vi "Prosilica Oscillating Exp.vi"() -> ()   [LabVIEW 2011]
uses:
  <vilib>/userDefined/High Color/IMAQdx.ctl
  <vilib>/vision/driver/IMAQdx.llb/IMAQdx Acquisition Mode.ctl
  <vilib>/vision/driver/IMAQdx.llb/IMAQdx Buffer Number Mode.ctl
  <vilib>/Platform/TimedLoop/XDataNode/timing_clust.ctl
  <vilib>/Platform/TimedLoop/XDataNode/nitl_modes.ctl
  <vilib>/Platform/TimedLoop/XDataNode/wakeup.ctl
  <vilib>/Platform/TimedLoop/XDataNode/XDataNode.xnode
  Program Files/National Instruments/LabVIEW 2011/resource/objmgr/imaqdx.rc
  <vilib>/vision/driver/NI_Vision_Acquisition_Software.lvlib
  Program Files/Mad City Labs/NanoDrive/Madlib.dll
  <vilib>/Platform/TimedLoop/XDataNode/XDNodeRunTimeDep.lvlib
panel:
  out "Starting Temperature":dbl
  out "Sample=Setpoints!":bool
  out "Waveform Chart":dbl(graph)
  out "Frames for Temp Ramp":dbl
  in  "Temp Setpoint":dbl=32.0 format="%.1f"
  in  "Time for Temp Ramp":dbl=1200.0 format="%<%H:%M>t"
  in  "Stop VI":bool
  in  "Start Acquisition":bool
  in  "Desired Z Position":dbl=100.0 min=0.0 max=200.0 step=0.1 format="%.4f"
  in  "Desired Y Position":dbl=100.0 min=0.0 max=200.0 step=0.1 format="%.4f"
  out "Current Z Position (um)":dbl format="%.2f"
  out "Current Y Position (um)":dbl format="%.2f"
  in  "Desire X Position":dbl=100.0 min=0.0 max=200.0 step=0.1 format="%.4f"
  out "Current X Position (um)":dbl format="%.2f"
  in  "Temp Control":bool
  in  "Frames to Temp Sample":dbl=100.0
  out "Current Temperature":dbl
  in  "VISA resource name selected":refnum<visa-resource-name>="COM3"
  in  "Path":path
  out "Frame Number":u32
  out "Frame Rate Out":dbl
  in  "Stop Acquisition":bool
  in  "Number of Frames":u32=18000
  in  "Frame Rate":dbl=5.0
  out "Image":T1(plugin-control)
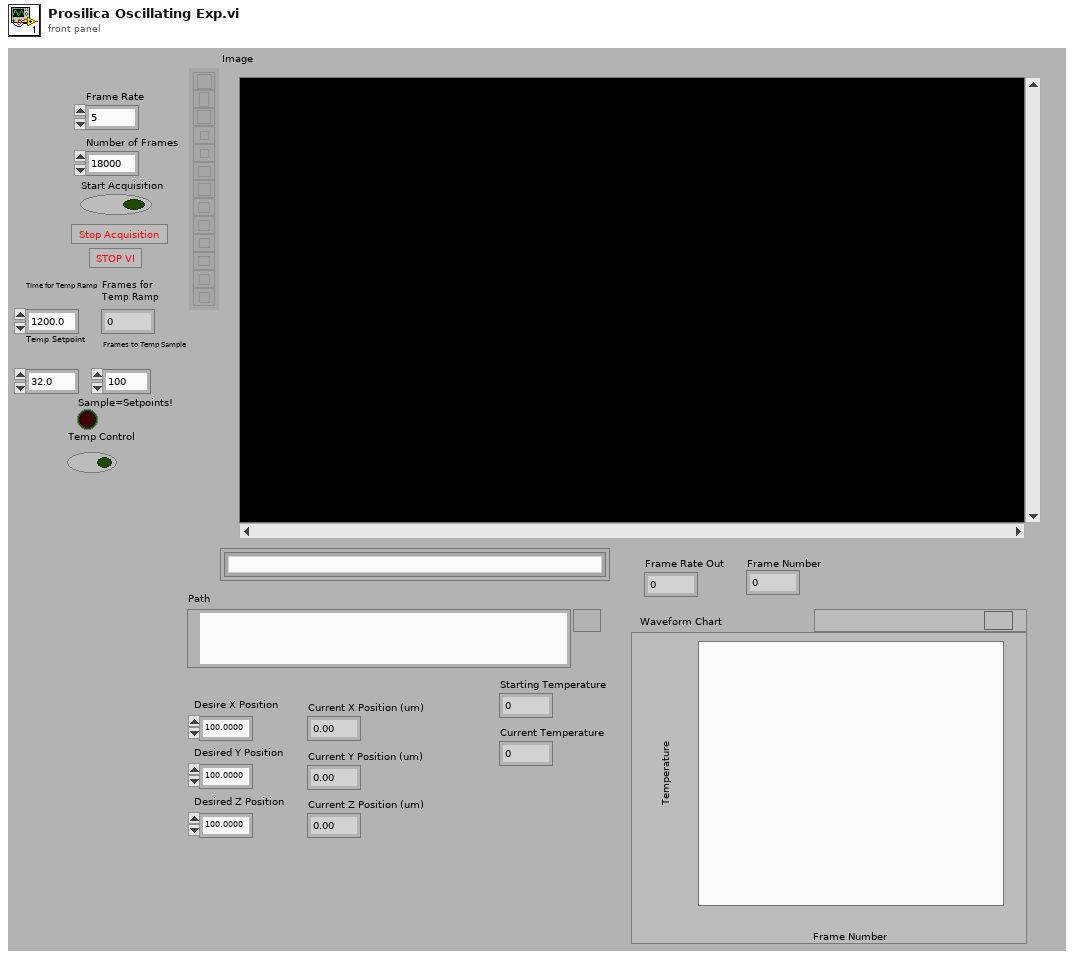
[diagram p1: front panel]
types:
  T1 = typedef "IMAQ Image.ctl" = refnum<image>
  T2 = typedef "IMAQdx.ctl" = refnum<k21>
  T3 = typedef "XDNodeRunTimeDep.lvlib/timing_clust.ctl" = cluster{"Expected End [f-1]":u64, "Actual End [f-1]":u64, "Finished Late? [f-1]":bool, "Expected End [i-1]":u64, "Actual End [i-1]":u64, "Finished Late? [i-1]":bool, "Expected Start [i]":u64, "Actual Start [i]":u64, "Expected Start [f]":u64, "Actual Start [f]":u64, "Source Name":string, "Structure Name":string, "Period":i64, "Deadline":i64, "Offset":i64, "Start":i64, "Priority":i32, "Timeout":i32, "Mode":T4, "Wakeup Reason":T5, "Error":errorcluster, "Source Type":string, "Secondary Source Type":string, "Global End Time":u64, "Global Start Time":u64, "Frame Duration":u64, "Iteration Duration":u64, "Assigned CPU":i32, "I/O Scan Engine Mode":u32}
  T4 = typedef "XDNodeRunTimeDep.lvlib/nitl_modes.ctl" = enum32{"No Change", "Process missed periods, maintain original phase", "Discard missed periods, maintain original phase", "Process missed periods, ignore original phase", "Discard missed periods, ignore original phase"}
  T5 = typedef "XDNodeRunTimeDep.lvlib/wakeup.ctl" = enum32{"Normal", "Aborted", "Asynchronous wakeup", "Timing source error", "Timed loop error", "Timeout"}
  T6 = typedef "NI_Vision_Acquisition_Software.lvlib/IMAQdx Acquisition Mode.ctl" = enum32{"One Shot", "Continuous"}
  T7 = typedef "NI_Vision_Acquisition_Software.lvlib/IMAQdx Buffer Number Mode.ctl" = enum32{"Next", "Last", "Buffer Number"}
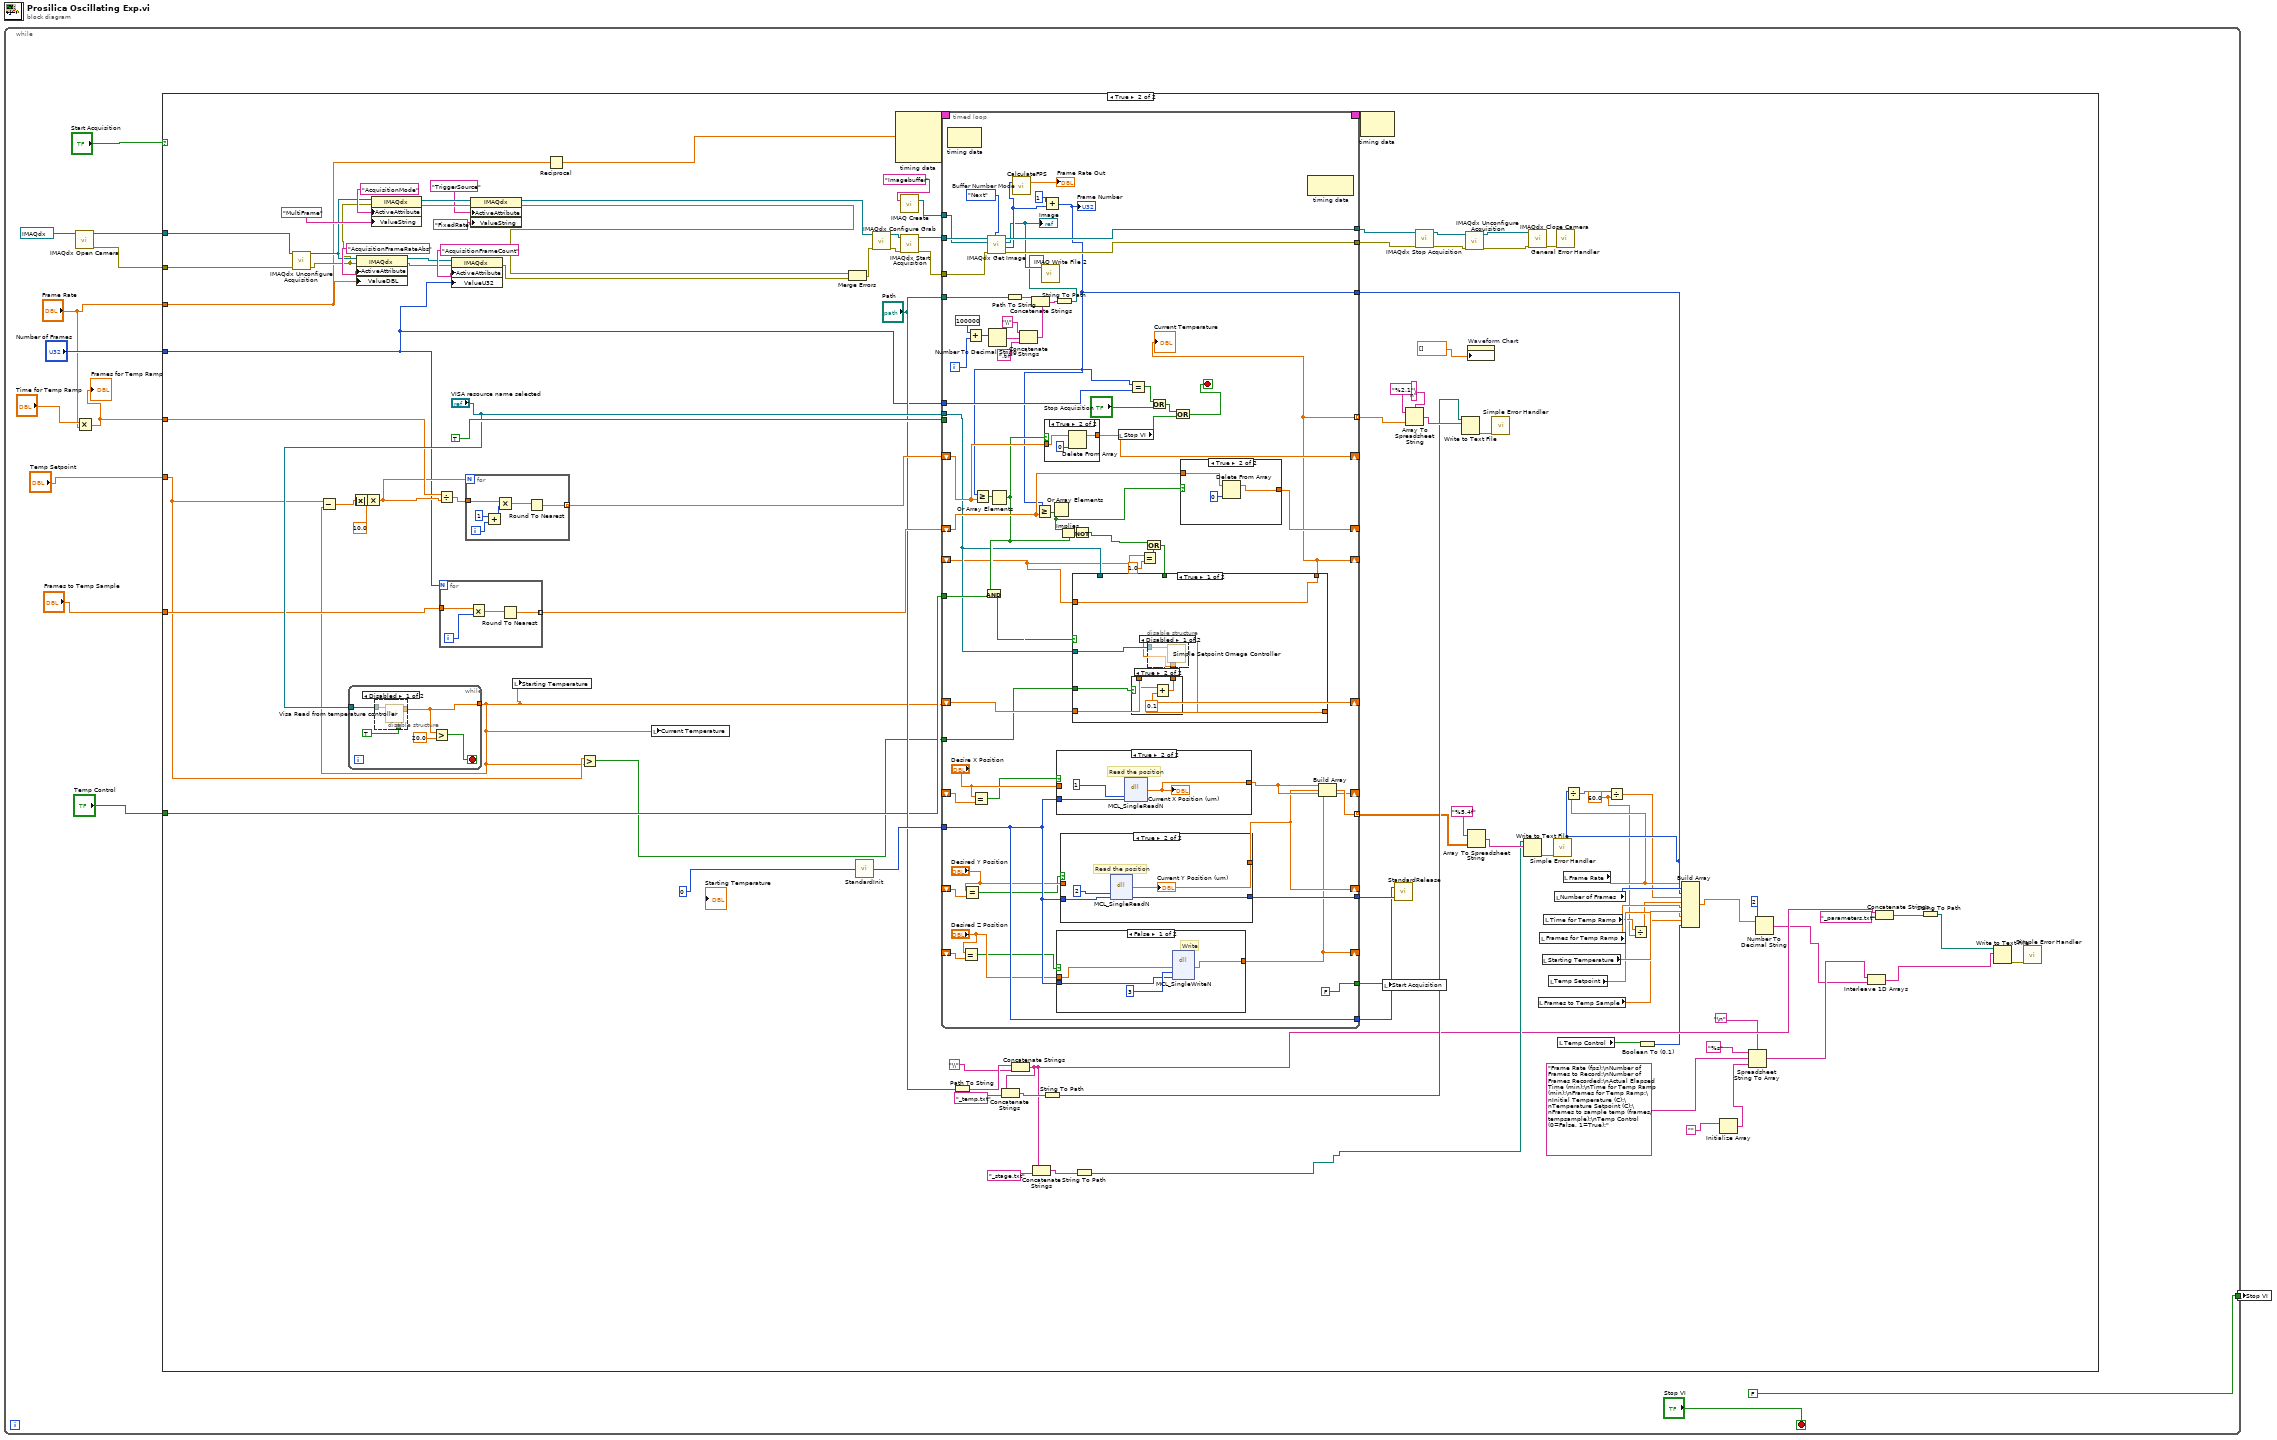
[diagram p0: block diagram]
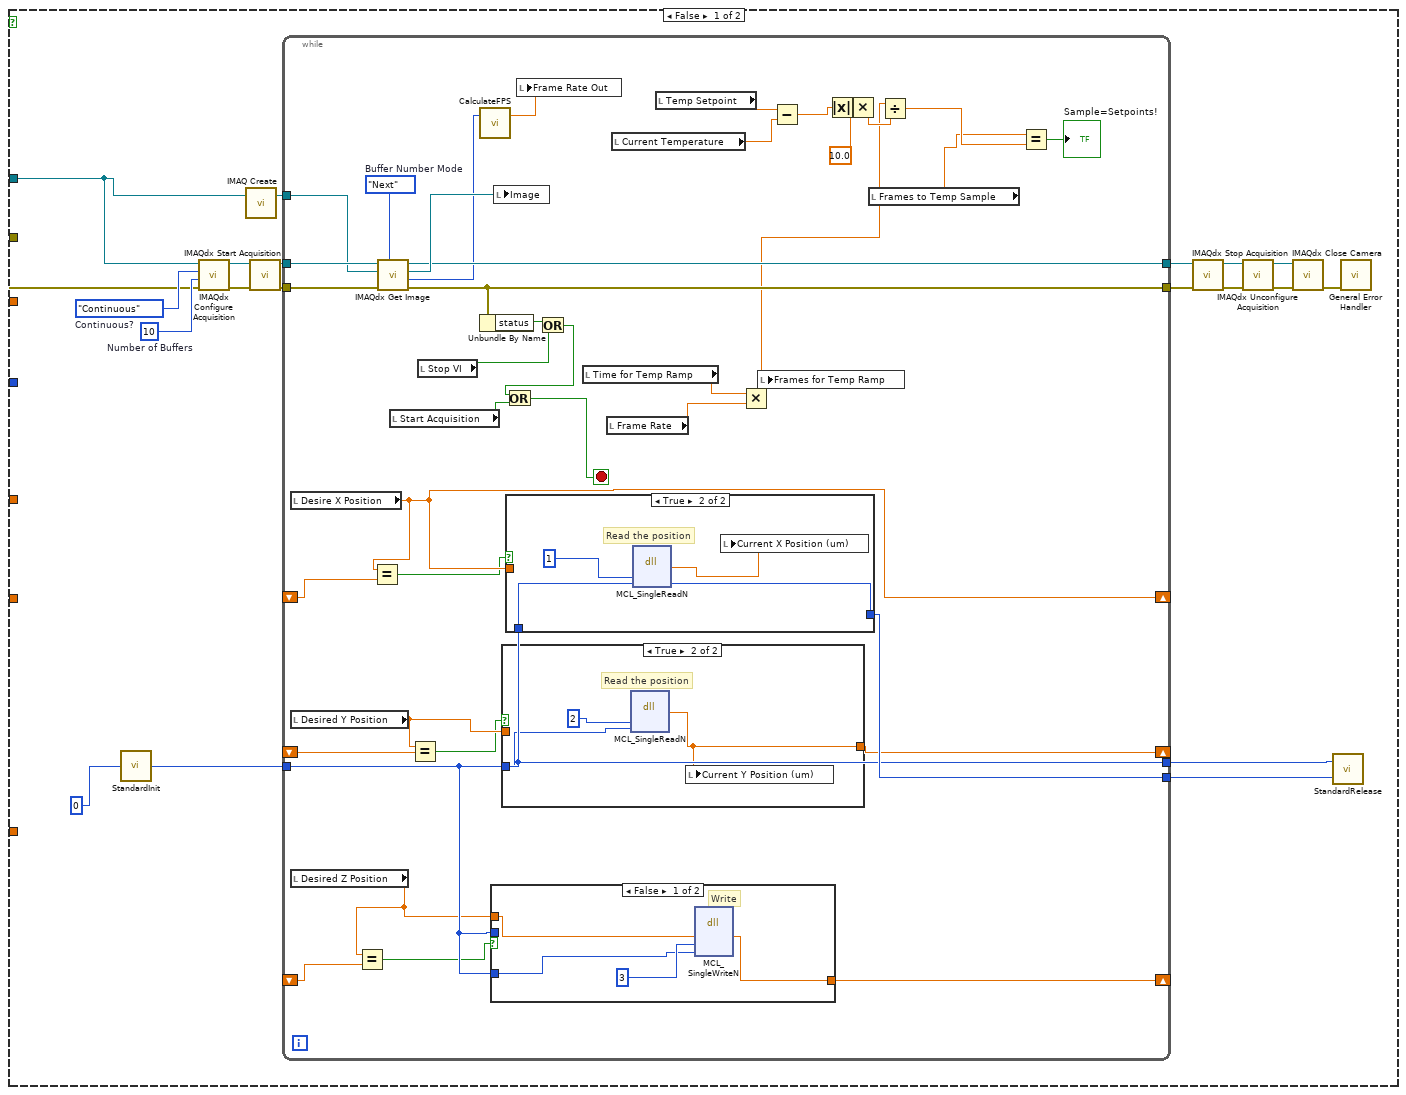
[diagram p2: hidden frame]
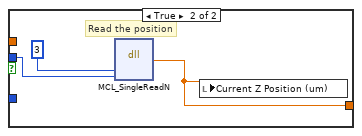
[diagram p3: hidden frame]
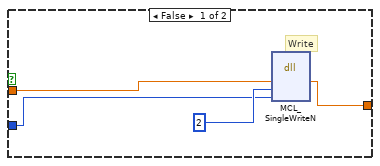
[diagram p4: hidden frame]
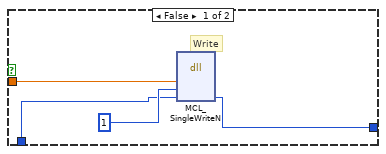
[diagram p5: hidden frame]
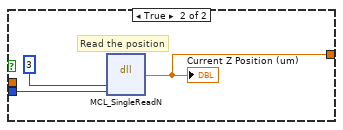
[diagram p6: hidden frame]
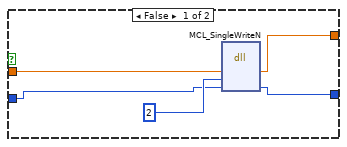
[diagram p7: hidden frame]
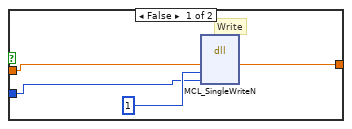
[diagram p8: hidden frame]
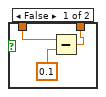
[diagram p12: hidden frame]
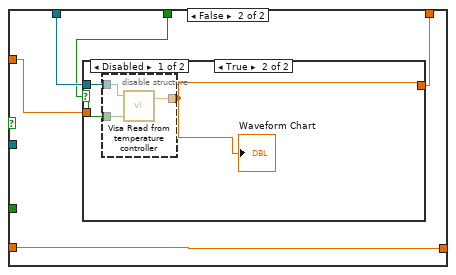
[diagram p13: hidden frame]
diagram:
  n1 = while {
    tunnel: [FALSE] -> w1
    stop <- "Stop VI" stop-if-true
    n2 = call <vilib>:"IMAQdx Open Camera.vi"("Session In"=T2 "cam0") -> ("error out"=w6:errorcluster, "Session Out"=w7:T2)  [unwired: 2 in, 7 out]
    n3 = Multiply(x="Time for Temp Ramp", y="Frame Rate") -> (x*y=w3:dbl)
    "Frames for Temp Ramp" <- w3
    n4 = case shown="True" "Start Acquisition" {
      tunnel: "Frame Rate" -> [_ w129]
      tunnel: "Number of Frames" -> [_ w132]
      tunnel: "Frames to Temp Sample" -> [_ w155]
      tunnel: "Temp Control" -> [_ w154]
      tunnel: w3 -> [_ w153]
      tunnel: w7 -> [w25 w152]
      tunnel: w6 -> [w24 w151]
      tunnel: "Temp Setpoint" -> [_ w135]
      frame False {
        w31 = IMAQdx_Acquisition_Mode."Continuous"  # Continuous?
        w30 = u32 10  # Number of Buffers
        n5 = call "StandardInit.vi"("Incoming Handle"=0) -> ("Outgoing Handle"=w17:i32)
        n6 = call <vilib>:"IMAQdx Configure Acquisition.vi"("error in"=w24, "Number of Buffers"=w30, "Continuous?"=w31, "Session In"=w25) -> ("error out"=w32:errorcluster, "Session Out"=w33:T2)  [unwired: 6 out]
        n7 = call "IMAQ Create"("Image Name"=w25) -> ("New Image"=w19:T1)  [unwired: 3 in, 2 out]
        n8 = call <vilib>:"IMAQdx Start Acquisition.vi"("error in"=w32, "Session In"=w33) -> ("error out"=w23:errorcluster, "Session Out"=w22:T2)  [unwired: 8 out]
        n9 = while {
          tunnel: w23 -> [w71]
          tunnel: w22 -> [w70]
          tunnel: [w67] -> w21
          tunnel: [w66] -> w20
          tunnel: w19 -> [w65]
          shift-right: [w58] -> _
          shift-left: _ -> [w59]
          tunnel: w17 -> [w53]
          tunnel: [w56] -> w16
          tunnel: [w53] -> w15
          shift-right: [w55] -> _
          shift-left: _ -> [w52]
          shift-right: [w54] -> _
          shift-left: _ -> [w49]
          stop <- w60 stop-if-true
          w72 = IMAQdx_Buffer_Number_Mode."Next"  # Buffer Number Mode
          n10 = local read "Desire X Position"() -> (w58:dbl)
          n11 = local read "Desired Y Position"() -> (w51:dbl)
          n12 = local read "Desired Z Position"() -> (w48:dbl)
          n13 = Equal?(x=w48, y=w49) -> (x = y?=w47:bool)
          n14 = Equal?(x=w58, y=w59) -> (x = y?=w57:bool)
          n15 = call <vilib>:"IMAQdx Get Image.vi"("Buffer Number Mode (Next)"=w72, "error in"=w71, "Image In"=w65, "Session In"=w70) -> ("error out"=w66:errorcluster, "Buffer Number Out"=w64:u32, "Image Out"=w69:T1, "Session Out"=w67:T2)  [unwired: 1 in, 3 out]
          n16 = local read "Start Acquisition"() -> (w62:bool)
          n17 = Equal?(x=w51, y=w52) -> (x = y?=w50:bool)
          n18 = local read "Stop VI"() -> (w63:bool)
          n19 = call "CalculateFPS.vi"("buffer number"=w64) -> ("acquired FPS"=w68:dbl)  [unwired: 2 out]
          n20 = Unbundle By Name(w66) -> ("status"=w73:bool)
          n21 = case shown="False" w47 {
            tunnel: w48 -> [w76 _]
            tunnel: [w75 w78] -> w54
            tunnel: w53 -> [w74 _]
            tunnel: w53 -> [_ w79]
            frame False {
              # "Write"
              n22 = dll-call lib="C:/Program Files/Mad City Labs/NanoDrive/Madlib.dll" fn="MCL_SingleWriteN"("position"=w76, "axis"=u32 3, "handle"=w74) -> ("position"=w75:dbl)  [unwired: 5 in, 3 out]
            }
            frame True {
              # "Read the position"
              n23 = dll-call lib="C:/Program Files/Mad City Labs/NanoDrive/Madlib.dll" fn="MCL_SingleReadN"("axis"=u32 3, "handle"=w79) -> (w78:dbl)  [unwired: 5 in, 2 out]
              n24 = local write "Current Z Position (um)"(w78) -> ()
            }
          }
          n25 = local write "Image"(w69) -> ()
          n26 = case shown="True" w50 {
            tunnel: [w83 w85] -> w55
            tunnel: w51 -> [w82 _]
            tunnel: w53 -> [w81 w86]
            frame False {
              # "Write"
              n27 = dll-call lib="C:/Program Files/Mad City Labs/NanoDrive/Madlib.dll" fn="MCL_SingleWriteN"("position"=w82, "axis"=u32 2, "handle"=w81) -> ("position"=w83:dbl)  [unwired: 5 in, 3 out]
            }
            frame True {
              # "Read the position"
              n28 = dll-call lib="C:/Program Files/Mad City Labs/NanoDrive/Madlib.dll" fn="MCL_SingleReadN"("axis"=u32 2, "handle"=w86) -> ("return type"=w85:dbl)  [unwired: 5 in, 2 out]
              n29 = local write "Current Y Position (um)"(w85) -> ()
            }
          }
          n30 = case shown="True" w57 {
            tunnel: w58 -> [w90 _]
            tunnel: w53 -> [w89 w93]
            tunnel: [w88 w92] -> w56
            frame False {
              # "Write"
              n31 = dll-call lib="C:/Program Files/Mad City Labs/NanoDrive/Madlib.dll" fn="MCL_SingleWriteN"("position"=w90, "axis"=u32 1, "handle"=w89) -> ("handle"=w88:i32)  [unwired: 5 in, 3 out]
            }
            frame True {
              # "Read the position"
              n32 = dll-call lib="C:/Program Files/Mad City Labs/NanoDrive/Madlib.dll" fn="MCL_SingleReadN"("axis"=u32 1, "handle"=w93) -> (w94:dbl, "handle"=w92:i32)  [unwired: 4 in, 2 out]
              n33 = local write "Current X Position (um)"(w94) -> ()
            }
          }
          n34 = local write "Frame Rate Out"(w68) -> ()
          n35 = Or(x=w73, y=w63) -> (x .or. y?=w61:bool)
          n36 = Or(x=w61, y=w62) -> (x .or. y?=w60:bool)
          n37 = local read "Time for Temp Ramp"() -> (w46:dbl)
          n38 = local read "Frame Rate"() -> (w45:dbl)
          n39 = local read "Current Temperature"() -> (w40:dbl)
          n40 = local read "Temp Setpoint"() -> (w41:dbl)
          n41 = Multiply(x=w46, y=w45) -> (x*y=w38:dbl)
          n42 = local write "Frames for Temp Ramp"(w38) -> ()
          n43 = Subtract(x=w41, y=w40) -> (x-y=w43:dbl)
          n44 = Absolute Value(x=w43) -> (abs(x)=w42:dbl)
          n45 = Multiply(x=w42, y=10.0) -> (x*y=w39:dbl)
          n46 = local read "Frames to Temp Sample"() -> (w36:dbl)
          n47 = Divide(x=w38, y=w39) -> (x/y=w37:dbl)
          n48 = Equal?(x=w36, y=w37) -> (x = y?=→"Sample=Setpoints!":bool)
        }
        n49 = call <vilib>:"IMAQdx Stop Acquisition.vi"("error in"=w20, "Session In"=w21) -> ("error out"=w26:errorcluster, "Session Out"=w27:T2)  [unwired: 8 out]
        n50 = call <vilib>:"IMAQdx Unconfigure Acquisition.vi"("error in"=w26, "Session In"=w27) -> ("error out"=w29:errorcluster, "Session Out"=w28:T2)  [unwired: 8 out]
        n51 = call <vilib>:"IMAQdx Close Camera.vi"("error in"=w29, "Session In"=w28) -> ("error out"=w34:errorcluster)  [unwired: 9 out]
        n52 = call "StandardRelease.vi"("Outgoing Handle"=w16, "Incoming Handle"=w15) -> ()  [unwired: 1 out]
        n53 = call <vilib>:"General Error Handler.vi"("error in (no error)"=w34) -> ()  [unwired: 1 in, 14 out]
      }
      frame True {
        w97 = 60.0 ("y")
        n54 = call <vilib>:"IMAQdx Unconfigure Acquisition.vi"("error in"=w151, "Session In"=w152) -> ("error out"=w172:errorcluster, "Session Out"=w183:T2)  [unwired: 8 out]
        n55 = while {
          tunnel: "VISA resource name selected" -> [w331]
          tunnel: [w329] -> w125
          stop <- w327 stop-if-true
          n56 = disable-structure shown="Disabled" {
            disable-tunnel: w331 -> [w334 _]
            disable-tunnel: TRUE -> [w333 _]
            disable-tunnel: [w332 _] -> w329
            frame Disabled {
              n57 = call <instrlib>:"Visa Read from temperature controller.vi"("run initialization of RS232"=w333, "VISA resource name selected"=w334) -> ("Temperature"=w332:dbl)  [unwired: 2 out]
            }
            frame Enabled {
            }
          }
          n58 = Greater?(x=w329, y=20.0) -> (0:w327:bool)
        }
        n59 = Subtract(x=w135, y=w125) -> (x-y=w137:dbl)
        n60 = Absolute Value(x=w137) -> (abs(x)=w136:dbl)
        n61 = property class="IMAQdx"(reference=w183, error in=w172, "ActiveAttribute"="AcquisitionFrameRateAbs", "ValueDBL"=w129) -> (reference out=w197:T2, error out=w196:errorcluster)
        n62 = Multiply(x=w136, y=10.0) -> (x*y=w134:dbl)
        n63 = property class="IMAQdx"(reference=w183, error in=w172, "ActiveAttribute"="AcquisitionMode", "ValueString"="MultiFrame") -> (reference out=w193:T2, error out=w192:errorcluster)
        n64 = Divide(x=w153, y=w134) -> (x/y=w171:dbl)
        n65 = for {
          N: w132 -> [_]
          tunnel: w155 -> [w338]
          tunnel: [w336] -> w169 mode=indexing
          i -> [w335]
          n66 = Multiply(x=w338, y=w335) -> (x*y=w337:dbl)
          n67 = Round To Nearest(number=w337) -> (nearest integer value=w336:dbl)
        }
        n68 = property class="IMAQdx"(reference=w197, error in=w196, "ActiveAttribute"="AcquisitionFrameCount", "ValueU32"=w132) -> (error out=w188:errorcluster)  [unwired: 1 out]
        n69 = for {
          N: w134 -> [_]
          tunnel: w171 -> [w344]
          tunnel: [w339] -> w170 mode=indexing
          i -> [w343]
          n70 = Add(x=1, y=w343) -> (x+y=w341:i32)
          n71 = Multiply(x=w344, y=w341) -> (x*y=w340:dbl)
          n72 = Round To Nearest(number=w340) -> (nearest integer value=w339:dbl)
        }
        n73 = property class="IMAQdx"(reference=w193, error in=w192, "ActiveAttribute"="TriggerSource", "ValueString"="FixedRate") -> (reference out=w189:T2, error out=w187:errorcluster)
        n74 = local write "Starting Temperature"(w125) -> ()
        n75 = Reciprocal(x=w129) -> (1/x=w128:dbl)
        n76 = Greater?(x=w135, y=w125) -> (0:w139:bool)
        n77 = local write "Current Temperature"(w125) -> ()
        n78 = Merge Errors(w187, w188) -> (w186:errorcluster)
        n79 = call "StandardInit.vi"("Incoming Handle"=0) -> ("Outgoing Handle"=w167:i32)
        n80 = call <vilib>:"IMAQdx Configure Grab.vi"("error in"=w186, "Session In"=w189) -> ("error out"=w145:errorcluster, "Session Out"=w146:T2)  [unwired: 8 out]
        n81 = node-c288(w128) -> (w131:T3)  [unwired: 3 out]
        n82 = call "IMAQ Create"("Image Name"="Imagebuffer") -> ("New Image"=w185:T1)  [unwired: 3 in, 2 out]
        n83 = call <vilib>:"IMAQdx Start Acquisition.vi"("error in"=w145, "Session In"=w146) -> ("error out"=w144:errorcluster, "Session Out"=w147:T2)  [unwired: 8 out]
        n84 = timed-loop {
          tunnel: w147 -> [w264]
          tunnel: w144 -> [w263]
          tunnel: w185 -> [w262]
          tunnel: [w260] -> w143
          tunnel: [w259] -> w142
          tunnel: "Path" -> [w251]
          tunnel: TRUE -> [_]
          tunnel: "VISA resource name selected" -> [w211]
          tunnel: [w210] -> w176 mode=indexing
          tunnel: w132 -> [w247]
          shift-right: [w210] -> _
          shift-left: _ -> [w208]
          shift-right: [w242] -> _
          shift-left: w125 -> [w243]
          tunnel: w154 -> [w239]
          tunnel: w139 -> [w238]
          tunnel: w167 -> [w236]
          tunnel: [w237] -> w166
          tunnel: [w236] -> w165
          tunnel: [w235] -> w157 mode=indexing
          shift-right: [w229] -> _
          shift-left: w169 -> [w230]
          shift-right: [w227] -> _
          shift-left: w170 -> [w228]
          tunnel: [FALSE] -> w148
          shift-right: [w223] -> _
          shift-left: _ -> [w222]
          shift-right: [w219] -> _
          shift-left: _ -> [w218]
          shift-right: [w215] -> _
          shift-left: _ -> [w214]
          timing: w131 -> [_]
          timing-out: [_] -> w130
          tunnel: [w200] -> w102
          i -> [w204]
          stop <- w232 stop-if-true
          w224 = IMAQdx_Buffer_Number_Mode."Next"  # Buffer Number Mode
          n85 = node-c288() -> ()  [unwired: 2 out]
          n86 = Equal?(x="Desired Z Position", y=w214) -> (x = y?=w212:bool)
          n87 = Equal?(x="Desired Y Position", y=w218) -> (x = y?=w216:bool)
          n88 = Add(x=100000, y=w204) -> (x+y=w202:i32)
          n89 = Equal?(x="Desire X Position", y=w222) -> (x = y?=w220:bool)
          n90 = call <vilib>:"IMAQdx Get Image.vi"("Buffer Number Mode (Next)"=w224, "error in"=w263, "Image In"=w262, "Session In"=w264) -> ("error out"=w259:errorcluster, "Buffer Number Out"=w258:u32, "Image Out"=w257:T1, "Session Out"=w260:T2)  [unwired: 1 in, 3 out]
          "Image" <- w257
          n91 = Number To Decimal String(number=w202) -> (decimal integer string=w254:string)  [unwired: 1 out]
          n92 = Path To String(path=w251) -> (string=w256:string)
          n93 = call "CalculateFPS.vi"("buffer number"=w258) -> ("acquired FPS"=→"Frame Rate Out":dbl)  [unwired: 2 out]
          n94 = Concatenate Strings("\\" ("string"), w254, ".tif") -> (w252:string)
          n95 = Concatenate Strings(w256, w252) -> (w255:string)
          n96 = Add(x=1, y=w258) -> (x+y=w200:u32)
          "Frame Number" <- w200
          n97 = Greater Or Equal?(x=w200, y=w228) -> (x >= y?=w245:bool[])
          n98 = Or Array Elements(Boolean array=w245) -> (logical OR=w226:bool)
          n99 = And(x=w226, y=w239) -> (x .and. y?=w240:bool)
          n100 = Greater Or Equal?(x=w200, y=w230) -> (x >= y?=w244:bool[])
          n101 = case shown="True" w226 {
            tunnel: w228 -> [w290 w292]
            tunnel: [w290 w291] -> w227
            frame False {
            }
            frame True {
              n102 = Delete From Array(array=w292, index=0) -> (array with subset deleted=w291:dbl[])  [unwired: 1 in, 1 out]
            }
          }
          n103 = Or Array Elements(Boolean array=w244) -> (logical OR=w231:bool)
          n104 = String To Path(string=w255) -> (path=w250:path)
          n105 = call-poly "IMAQ Write File 2"("File Path"=w250, "Image"=w257) -> ()  [unwired: 3 in, 7 out]
          n106 = case shown="True" w220 {
            tunnel: w236 -> [w284 w289]
            tunnel: [w283 w288] -> w223
            tunnel: "Desire X Position" -> [w285 _]
            frame False {
              # "Write"
              n107 = dll-call lib="C:/Program Files/Mad City Labs/NanoDrive/Madlib.dll" fn="MCL_SingleWriteN"("position"=w285, "axis"=u32 1, "handle"=w284) -> ("position"=w283:dbl)  [unwired: 5 in, 3 out]
            }
            frame True {
              # "Read the position"
              n108 = dll-call lib="C:/Program Files/Mad City Labs/NanoDrive/Madlib.dll" fn="MCL_SingleReadN"("axis"=u32 1, "handle"=w289) -> (w288:dbl)  [unwired: 5 in, 2 out]
              "Current X Position (um)" <- w288
            }
          }
          n109 = case shown="False" w212 {
            tunnel: w236 -> [w267 w273]
            tunnel: [w268 w272] -> w215
            tunnel: "Desired Z Position" -> [w269 _]
            frame False {
              # "Write"
              n110 = dll-call lib="C:/Program Files/Mad City Labs/NanoDrive/Madlib.dll" fn="MCL_SingleWriteN"("position"=w269, "axis"=u32 3, "handle"=w267) -> ("position"=w268:dbl)  [unwired: 5 in, 3 out]
            }
            frame True {
              # "Read the position"
              n111 = dll-call lib="C:/Program Files/Mad City Labs/NanoDrive/Madlib.dll" fn="MCL_SingleReadN"("axis"=u32 3, "handle"=w273) -> (w272:dbl)  [unwired: 5 in, 2 out]
              "Current Z Position (um)" <- w272
            }
          }
          n112 = Implies(1:w226, 2:w231) -> (0:w241:bool)
          n113 = case shown="True" w216 {
            tunnel: [w274 w282] -> w237
            tunnel: w236 -> [w276 w281]
            tunnel: [w275 w280] -> w219
            tunnel: "Desired Y Position" -> [w277 _]
            frame False {
              n114 = dll-call lib="C:/Program Files/Mad City Labs/NanoDrive/Madlib.dll" fn="MCL_SingleWriteN"("position"=w277, "axis"=u32 2, "handle"=w276) -> ("position"=w275:dbl, "handle"=w274:i32)  [unwired: 4 in, 3 out]
            }
            frame True {
              # "Read the position"
              n115 = dll-call lib="C:/Program Files/Mad City Labs/NanoDrive/Madlib.dll" fn="MCL_SingleReadN"("axis"=u32 2, "handle"=w281) -> (w280:dbl, "handle"=w282:i32)  [unwired: 4 in, 2 out]
              "Current Y Position (um)" <- w280
            }
          }
          n116 = Not(x=w241) -> (.not. x?=w209:bool)
          n117 = local read "Stop VI"() -> (w233:bool)
          n118 = Equal?(x=w200, y=w247) -> (x = y?=w246:bool)
          n119 = Equal?(x=w208, y=1.0) -> (x = y?=w206:bool)
          n120 = Or(x=w209, y=w206) -> (x .or. y?=w205:bool)
          n121 = case shown="True" w240 {
            tunnel: w211 -> [w302 _]
            tunnel: w243 -> [w301 w315]
            tunnel: [w300 w315] -> w242
            tunnel: w238 -> [w299 _]
            tunnel: w211 -> [_ w314]
            tunnel: [w298 w313] -> w210
            tunnel: w208 -> [w298 w312]
            tunnel: w205 -> [_ w311]
            frame True {
              n122 = case shown="True" w299 {
                tunnel: w301 -> [w306 w309]
                tunnel: [w305 w308] -> w300
                frame False {
                  n123 = Subtract(x=w306, y=0.1) -> (x-y=w305:dbl)
                }
                frame True {
                  n124 = Add(x=w309, y=0.1) -> (x+y=w308:dbl)
                }
              }
              n125 = disable-structure shown="Disabled" {
                disable-tunnel: w302 -> [w304 _]
                disable-tunnel: w300 -> [w303 _]
                frame Disabled {
                  n126 = call "Simple Setpoint Omega Controller.vi"("Set Point Temperature"=w303, "VISA resource name"=w304) -> ()  [unwired: 10 out]
                }
                frame Enabled {
                }
              }
            }
            frame False {
              n127 = case shown="True" w311 {
                selector: w311 -> [_ w319]
                tunnel: w314 -> [_ w318]
                tunnel: [w316 w317] -> w313
                tunnel: w312 -> [w316 _]
                frame False {
                }
                frame True {
                  n128 = disable-structure shown="Disabled" {
                    disable-tunnel: w319 -> [w322 _]
                    disable-tunnel: w318 -> [w321 _]
                    disable-tunnel: [w320 _] -> w317
                    frame Disabled {
                      n129 = call <instrlib>:"Visa Read from temperature controller.vi"("run initialization of RS232"=w322, "VISA resource name selected"=w321) -> ("Temperature"=w320:dbl)  [unwired: 2 out]
                    }
                    frame Enabled {
                    }
                  }
                  "Waveform Chart" <- w317
                }
              }
            }
          }
          "Current Temperature" <- w210
          n130 = Or(x=w246, y="Stop Acquisition") -> (x .or. y?=w234:bool)
          n131 = Or(x=w234, y=w233) -> (x .or. y?=w232:bool)
          n132 = case shown="True" w231 {
            tunnel: w230 -> [w294 w297]
            tunnel: [w294 w295] -> w229
            frame False {
            }
            frame True {
              n133 = Delete From Array(array=w297, index=0) -> (array with subset deleted=w295:dbl[])  [unwired: 1 in, 1 out]
            }
          }
          n134 = node-c288() -> ()  [unwired: 2 out]
          n135 = Build Array(w223, w219, w215) -> (w235:dbl[])
        }
        n136 = Path To String(path="Path") -> (string=w127:string)
        n137 = Concatenate Strings(w127, "\\" ("string")) -> (w124:string)
        n138 = Concatenate Strings(w124, "_temp.txt") -> (w175:string)
        n139 = Concatenate Strings(w124, "_stage.txt") -> (w163:string)
        n140 = String To Path(string=w175) -> (path=w173:path)
        n141 = String To Path(string=w163) -> (path=w156:path)
        n142 = node-c288(w130) -> ()  [unwired: 1 out]
        n143 = local write "Start Acquisition"(w148) -> ()
        n144 = call "StandardRelease.vi"("Outgoing Handle"=w166, "Incoming Handle"=w165) -> ()  [unwired: 1 out]
        n145 = Array To Spreadsheet String(delimiter (Tab)="\n", array=w176, 3:"%2.1f") -> (spreadsheet string=w179:string)
        n146 = call <vilib>:"IMAQdx Stop Acquisition.vi"("error in"=w142, "Session In"=w143) -> ("error out"=w140:errorcluster, "Session Out"=w141:T2)  [unwired: 8 out]
        n147 = Write to Text File(file (use dialog)=w173, text=w179) -> (error out=w180:errorcluster)  [unwired: 1 in, 3 out]
        n148 = call <vilib>:"IMAQdx Unconfigure Acquisition.vi"("error in"=w140, "Session In"=w141) -> ("error out"=w149:errorcluster, "Session Out"=w150:T2)  [unwired: 8 out]
        n149 = Array To Spreadsheet String(array=w157, 3:"%5.4f") -> (spreadsheet string=w158:string)  [unwired: 1 out]
        n150 = property on="Waveform Chart" class="WFChart (strict)"("History Data"=dbl[] []) -> ()  [unwired: 2 in, 2 out]
        n151 = call <vilib>:"Simple Error Handler.vi"("error in (no error)"=w180) -> ()  [unwired: 1 in, 8 out]
        n152 = Write to Text File(file (use dialog)=w156, text=w158) -> (error out=w159:errorcluster)  [unwired: 1 in, 3 out]
        n153 = call <vilib>:"IMAQdx Close Camera.vi"("error in"=w149, "Session In"=w150) -> ("error out"=w182:errorcluster)  [unwired: 9 out]
        n154 = local read "Frames to Temp Sample"() -> (w116:dbl)
        n155 = local read "Frames for Temp Ramp"() -> (w119:dbl)
        n156 = local read "Starting Temperature"() -> (w118:dbl)
        n157 = local read "Time for Temp Ramp"() -> (w98:dbl)
        n158 = local read "Temp Setpoint"() -> (w117:dbl)
        n159 = call <vilib>:"Simple Error Handler.vi"("error in (no error)"=w159) -> ()  [unwired: 1 in, 8 out]
        n160 = local read "Number of Frames"() -> (w120:u32)
        n161 = call <vilib>:"General Error Handler.vi"("error in (no error)"=w182) -> ()  [unwired: 1 in, 14 out]
        n162 = local read "Temp Control"() -> (w115:bool)
        n163 = local read "Frame Rate"() -> (w101:dbl)
        n164 = Divide(x=w102, y=w101) -> (x/y=w100:fxp<+/-,24,11>)
        n165 = Divide(x=w100, y=w97) -> (x/y=w99:dbl)
        n166 = Divide(x=w98, y=w97) -> (x/y=w96:dbl)
        n167 = Boolean To (0,1)(Boolean=w115) -> (0, 1=w114:i16)
        n168 = Build Array(w101, w120, w102, w99, w96, w119, w118, w117, w116, w114) -> (w108:dbl[])
        n169 = Initialize Array("") -> (w111:string[])  [unwired: 1 out]
        n170 = Spreadsheet String To Array(delimiter (Tab)="\n", format string="%s", spreadsheet string="Frame Rate (fps):\nNumber of Frames to Record:\nNumber of Frames Recorded:\nActual Elapsed Time (min):\nTime for Temp Ramp (min):\nFrames for Temp Ramp:\nInitial Temperature (C):\nTemperature Setpoint (C):\nFrames to sample temp (frames/tempsample):\nTemp Control (0=False, 1=True):", array type (2D Dbl)=w111) -> (array=w106:string[])
        n171 = Number To Decimal String(number=w108, width (-)=i16 2) -> (decimal integer string=w105:string[])
        n172 = Interleave 1D Arrays(w106, w105) -> (w121:string[])
        n173 = Concatenate Strings(w124, "_parameters.txt" ("string")) -> (w103:string)
        n174 = String To Path(string=w103) -> (path=w122:path)
        n175 = Write to Text File(file (use dialog)=w122, text=w121) -> (error out=w123:errorcluster)  [unwired: 1 in, 3 out]
        n176 = call <vilib>:"Simple Error Handler.vi"("error in (no error)"=w123) -> ()  [unwired: 1 in, 8 out]
      }
    }
  }
  n177 = local write "Stop VI"(w1) -> ()
